vi "WD_Set_NULL.vi"(8 "error in (no error)":errorcluster, 10 "Workplace_id":i16, 11 "DBlink":string="Driver={ODBC Driver 17 for SQL Server};Server=localhost\\SQLEXPRESS;Database=ZDX201;UID=labview;PWD=Dsa@54137926") -> (0 "error out":errorcluster, 2 "Workplace: assemble":cluster{"條碼A":string, "條碼B":string}[](array[cluster]))   [LabVIEW 2019]
uses:
  <vilib>/addons/database/Connection.llb/DB Tools Open Connec (String).vi
  <vilib>/addons/database/Connection.llb/Conn Execute.vi
  <vilib>/addons/database/Recordset.llb/Rec Fetch Recordset Data (R).vi
  <vilib>/addons/database/Recordset.llb/Rec Destroy - Connection.vi
  <vilib>/addons/database/_DB Variant To Data/Database Variant To Data.xnode
  <vilib>/addons/database/NI_Database_API.lvlib
panel:
  out "查詢結果":string="Update [workplace_data] \nset  \n[barcode A] = NULL       \n  ,[barcode B] = NULL\n"
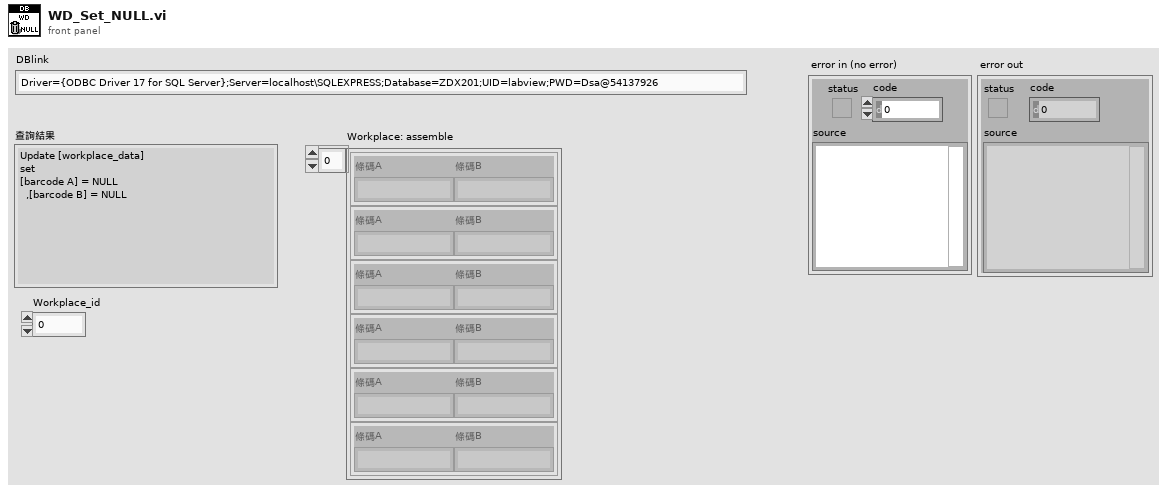
[diagram p1: front panel]
types:
  T1 = typedef "NI_Database_API.lvlib/Conn ObjectReference.ctl" = refnum<k1>
  T2 = typedef "NI_Database_API.lvlib/Rec ObjectReference.ctl" = refnum<k1>
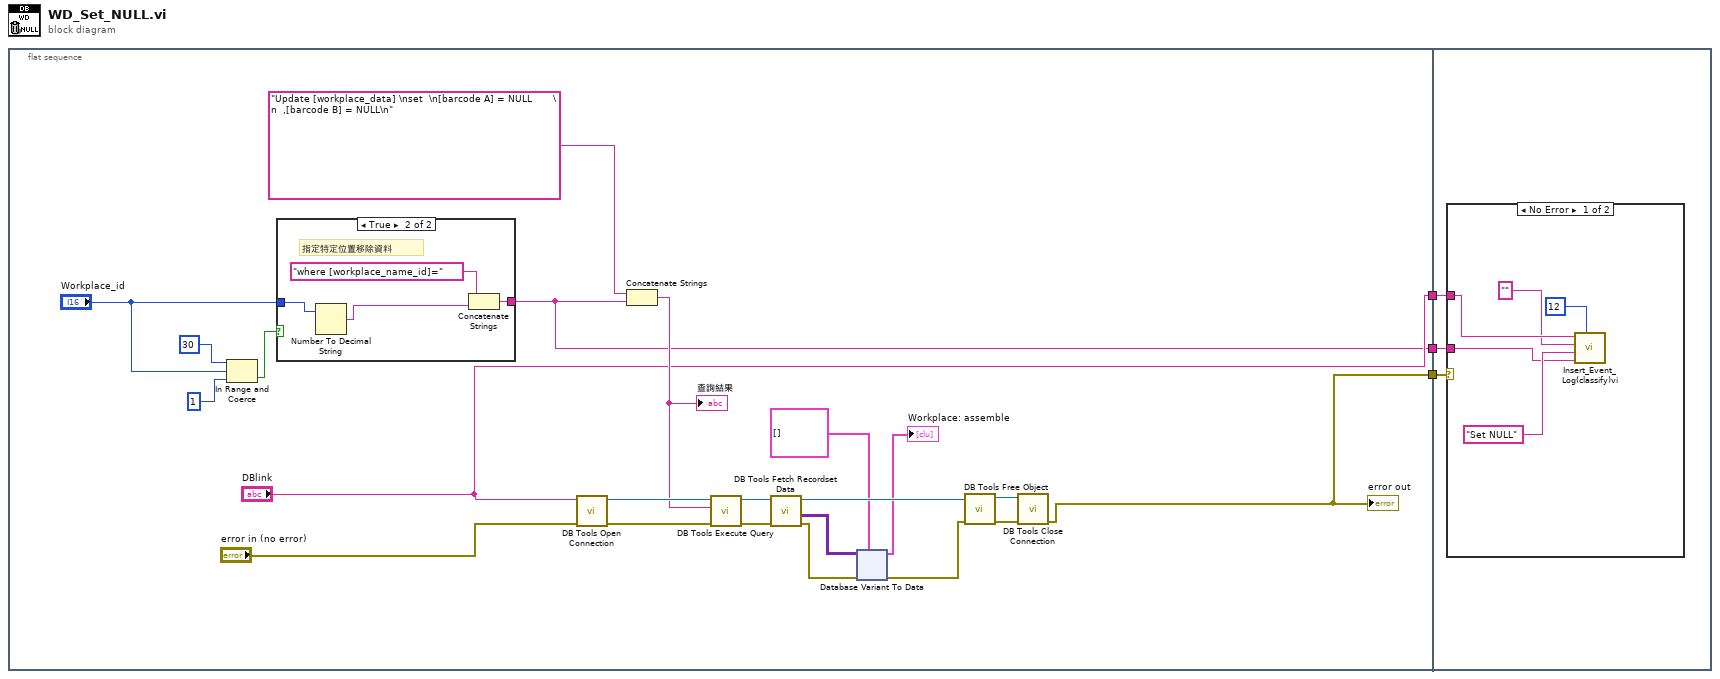
[diagram p0: block diagram]
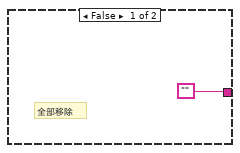
[diagram p2: hidden frame]
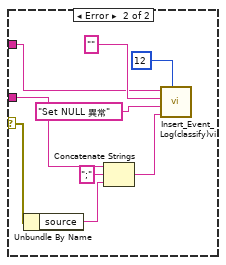
[diagram p3: hidden frame]
diagram:
  n1 = flat-sequence {
    tunnel: [w6] -> w3
    tunnel: ["DBlink"] -> w2
    tunnel: [w4] -> w1
    tunnel: w3 -> [w105]
    tunnel: w2 -> [w104]
    tunnel: w1 -> [w103]
    frame #0 {
      n2 = In Range and Coerce(upper limit=i16 30, x="Workplace_id", lower limit=i16 1) -> (In Range?=w10:bool)  [unwired: 1 out]
      n3 = case shown="True" w10 {
        tunnel: "Workplace_id" -> [_ w30]
        tunnel: ["" w27] -> w4
        frame False {
          # "全部移除"
        }
        frame True {
          # "指定特定位置移除資料"
          n4 = Number To Decimal String(number=w30) -> (decimal integer string=w28:string)  [unwired: 1 in]
          n5 = Concatenate Strings("where [workplace_name_id]=", w28) -> (w27:string)
        }
      }
      n6 = call-poly <vilib>:"DB Tools Open Connection.vi"("error in (no error)"="error in (no error)", "connection information"="DBlink") -> ("error out"=w25:errorcluster, "connection reference"=w24:T1)  [unwired: 6 in]
      n7 = Concatenate Strings("Update [workplace_data] \nset  \n[barcode A] = NULL       \n  ,[barcode B] = NULL\n", w4) -> (w7:string)
      "查詢結果" <- w7
      n8 = call-poly <vilib>:"DB Tools Execute Query.vi"("error in (no error)"=w25, "SQL query"=w7, "connection reference"=w24) -> ("error out"=w22:errorcluster, "recordset reference"=w23:T2)  [unwired: 5 in]
      n9 = call-poly <vilib>:"DB Tools Fetch Recordset Data.vi"("error in (no error)"=w22, "recordset reference"=w23) -> ("error out"=w17:errorcluster, "recordset data"=w16:variant[][], "recordset reference out"=w18:T2)  [unwired: 3 in]
      n10 = xnode "Database Variant To Data"("database variant"=w16, "error in (no error)"=w17, "type"=cluster{"條碼A":string, "條碼B":string}[] [] ("Workplace: assemble")) -> ("data"=→"Workplace: assemble":cluster{"條碼A":string, "條碼B":string}[], "error out"=w19:errorcluster)
      n11 = call-poly <vilib>:"DB Tools Free Object.vi"("error in (no error)"=w19, "recordset reference"=w18) -> ("error out"=w20:errorcluster, "connection reference"=w21:T1)  [unwired: 8 in]
      n12 = call <vilib>:"DB Tools Close Connection.vi"("error in (no error)"=w20, "connection reference"=w21) -> ("error out"=w6:errorcluster)  [unwired: 5 in]
      "error out" <- w6
    }
    frame #1 {
      n13 = case shown="No Error" w105 {
        selector: w105 -> [_ w113]
        tunnel: w104 -> [w110 w116]
        tunnel: w103 -> [w107 w115]
        frame No Error {
          n14 = call "Insert_Event_Log(classify)vi.vi"("classify"=i16 12, "data"=w107, "message"="Set NULL", "id"="", "DBlink"=w110) -> ()  [unwired: 6 in, 1 out]
        }
        frame Error {
          n15 = Unbundle By Name(w113) -> ("source"=w112:string)
          n16 = Concatenate Strings(w115, ";" ("string"), w112) -> (w111:string)
          n17 = call "Insert_Event_Log(classify)vi.vi"("classify"=i16 12, "data"=w111, "message"="Set NULL 異常", "id"="", "DBlink"=w116) -> ()  [unwired: 6 in, 1 out]
        }
      }
    }
  }
